vi "Partition_Sort.vi"(8 "FreezeIdx":i32[](array[numeric]), 9 "PartitionArray":string[](array[string]), 10 "FreezeTemps":dbl[](array[numeric]), 11 "Temps":dbl[][](array[numeric])) -> (0 "Freeze Idx / Part Array":i32[][](array[numeric]), 1 "Freeze / Part Array":bool[][](array[boolean]), 2 "FreezeTenos / Part Array":dbl[][](array[numeric]), 3 "MaxSize":i32)   [LabVIEW 2022 SP3]
uses:
  162fd0d4-48cb-478f-89f4-36ef44532280.vi
  <vilib>/Comparison/Less/Less Functor/Less Functor.lvclass
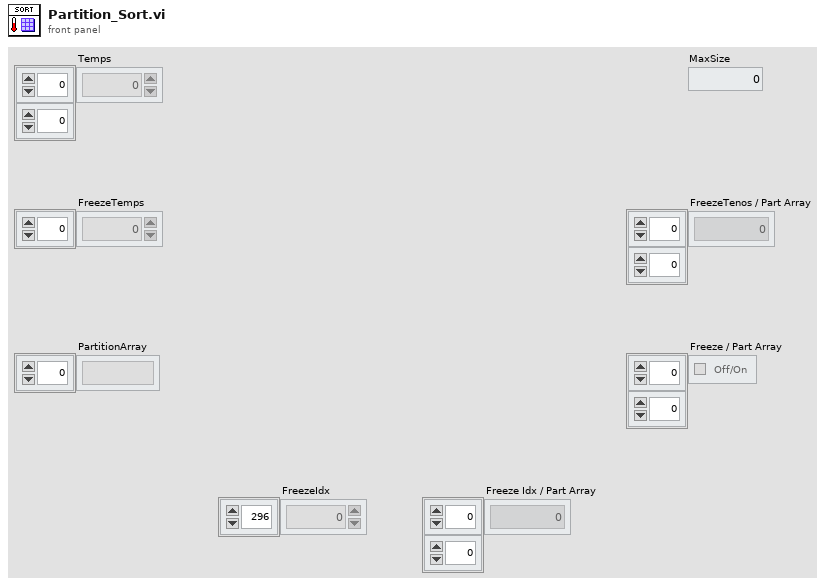
[diagram p1: front panel]
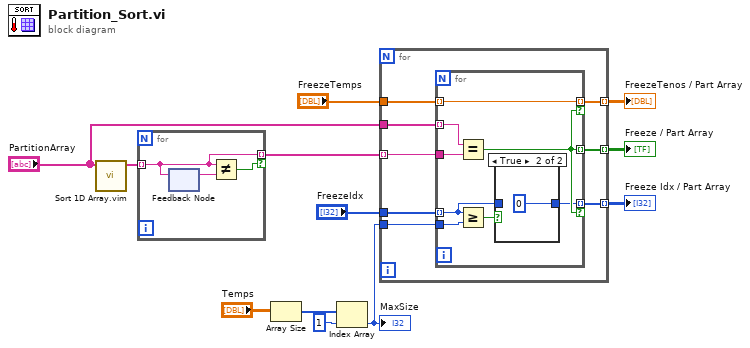
[diagram p0: block diagram]
diagram:
  n1 = call "Sort 1D Array.vim"("unsorted array"="PartitionArray") -> ("sorted array"=w3:string[])  [unwired: 10 in]
  n2 = for {
    tunnel: w3 -> [w13] mode=indexing
    tunnel: [w13] -> w4 mode=indexing if=w15
    n3 = feedback-in #1(w13) -> ()
    n4 = feedback #1() -> (w14:string)  [unwired: 1 in]
    n5 = Not Equal?(x=w13, y=w14) -> (x != y?=w15:bool)
  }
  n6 = Array Size(array="Temps") -> (size(s)=w10:i32[])
  n7 = Index Array(array=w10, index=1) -> (element=w1:i32)
  "MaxSize" <- w1
  n8 = for {
    tunnel: "PartitionArray" -> [w23]
    tunnel: "FreezeTemps" -> [w22]
    tunnel: w4 -> [w21] mode=indexing
    tunnel: [w20] -> w5 mode=indexing
    tunnel: [w19] -> w6 mode=indexing
    tunnel: "FreezeIdx" -> [w18]
    tunnel: [w17] -> w12 mode=indexing
    tunnel: w1 -> [w16]
    n9 = for {
      tunnel: w23 -> [w31] mode=indexing
      tunnel: w22 -> [w29] mode=indexing
      tunnel: w21 -> [w30]
      tunnel: [w29] -> w20 mode=indexing if=w28
      tunnel: [w28] -> w19 mode=indexing
      tunnel: w18 -> [w27] mode=indexing
      tunnel: [w24] -> w17 mode=indexing if=w28
      tunnel: w16 -> [w26]
      n10 = Equal?(x=w31, y=w30) -> (x = y?=w28:bool)
      n11 = Greater Or Equal?(x=w27, y=w26) -> (x >= y?=w25:bool)
      n12 = case shown="True" w25 {
        tunnel: w27 -> [w32 _]
        tunnel: [w32 0] -> w24
        frame False {
        }
        frame True {
        }
      }
    }
  }
  "Freeze Idx / Part Array" <- w12
  "Freeze / Part Array" <- w6
  "FreezeTenos / Part Array" <- w5
